vi "Configure Stamps.vi"(7 "Config Manager in":refnum<class "Config Manager Class.lvclass">, 8 "error in":errorcluster, 11 "WorkTable in":refnum<class "WorkTable Class.lvclass">) -> (0 "error out":errorcluster, 3 "WorkTable out":refnum<class "WorkTable Class.lvclass">)   [LabVIEW 2011, in "WorkTable Class.lvclass"]
uses:
  WorkTable Class.lvclass
  Config Manager Class/Config Manager Class.lvclass
  Config Manager Class/Type Definitions/Manifold Channel Types.ctl
  Type Definitions/Worktable_Stamps.ctl
  Type Definitions/Worktable_Stamp.ctl
  Utils/Type Definitions/Position_Orientation.ctl
  Vec3d Class/Vec3d Class.lvclass
  Orient3d Class/Orient3d Class.lvclass
  Config Manager Class/Type Definitions/Stamp Type.ctl
  Config Manager Class/Read Manifold Channel Other.vi
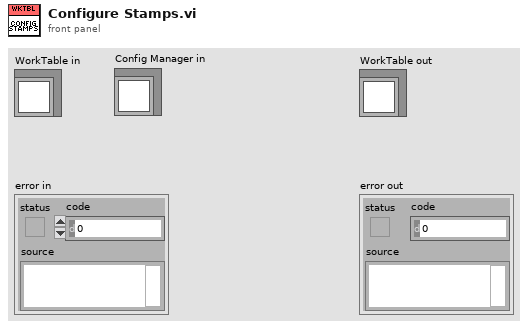
[diagram p1: front panel]
types:
  T1 = typedef "Manifold Channel Types.ctl" = enum16{"GANTRY_HEAD_OUTER", "GANTRY_HEAD_INNER", "GLUE_RESERVOIR_CHUCK", "STAMP_TOOL_CHUCK", "WEIGHT_TOOL_CHUCK"}
  T2 = typedef "Worktable_Stamps.ctl" = cluster{"Stamp Slots":T3[], "Vacuum Channel":i32}
  T3 = typedef "Worktable_Stamp.ctl" = cluster{"Stamp State":enum16{"Empty", "Populated", "Used"}, "Location/Orientation":T4, "Stamp Type":T5}
  T4 = typedef "Position_Orientation.ctl" = cluster{"Center":refnum<class "Vec3d Class.lvclass">, "Orientation":refnum<class "Orient3d Class.lvclass">}
  T5 = typedef "Stamp Type.ctl" = enum16{"Stamp 1", "Stamp 2", "Stamp 3", "Stamp 4", "Stamp 5"}
  T6 = typedef "Part Type.ctl" = enum16{"BBM", "HDI", "BARE HDI", "GLUERESERVOIR", "STAMP_1", "STAMP_2", "STAMP_3", "STAMP_4", "STAMP_5", "WEIGHT_1", "WEIGHT_2", "WEIGHT_3", "WEIGHT_4", "WEIGHT_5", "WEIGHT_6", "WEIGHT_7", "WEIGHT_8", "PICKER_TOOL", "GRABER_TOOL"}
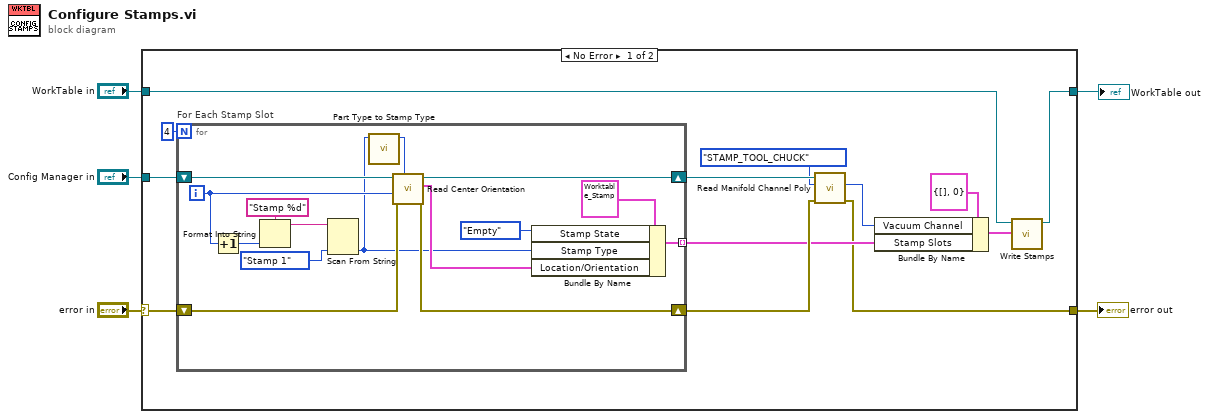
[diagram p0: block diagram]
diagram:
  n1 = case shown="No Error" "error in" {
    selector: "error in" -> [w12 w35]
    tunnel: [w6 w35] -> w2
    tunnel: [w17 w34] -> w3
    tunnel: "WorkTable in" -> [w18 w34]
    tunnel: "Config Manager in" -> [w13 _]
    frame No Error {
      n2 = for "For Each Stamp Slot" {
        N: 4 ("dimension size") -> [_]
        tunnel: [w33] -> w8 mode=indexing
        shift-right: [w26] -> w9
        shift-left: w12 -> [w27]
        shift-right: [w28] -> w11
        shift-left: w13 -> [w30]
        i -> [w25]
        n3 = Increment(x=w25) -> (x+1=w24:i32)
        n4 = Format Into String(format string="Stamp %d", w24) -> (resulting string=w22:string)  [unwired: 2 in, 1 out]
        n5 = Scan From String(input string=w22, default 1=Stamp_Type."Stamp 1" ("Stamp Type")) -> (output 1=w20:T5)  [unwired: 3 in, 3 out]
        n6 = call "Part Type to Stamp Type.vi"("Stamp Type"=w20) -> ("Part Type"=w19:T6)  [unwired: 9 in, 1 out]
        n7 = call "Read Center Orientation.vi"("Part Type"=w19, "error in"=w27, "slot"=w25, "Config Manager in"=w30) -> ("error out"=w26:errorcluster, "Location/Orientation"=w29:T4, "Config Manager out"=w28:refnum<class "Config Manager Class.lvclass">)  [unwired: 5 in]
        n8 = Bundle By Name(cluster=T3 {"Stamp State"=enum."Empty", "Location/Orientation"={"Center"=refnum, "Orientation"=refnum}, "Stamp Type"=enum."Stamp 1"} ("Stamp Slot"), "Stamp State"=enum16{"Empty", "Populated", "Used"}."Empty", "Stamp Type"=w20, "Location/Orientation"=w29) -> (w33:T3)
      }
      n9 = call-poly "Read Manifold Channel Poly.vi"("error in"=w9, "Manifold Channel Type"=Manifold_Channel_Types."STAMP_TOOL_CHUCK", "Config Manager in"=w11) -> ("error out"=w6:errorcluster, "Channel"=w7:i32)  [unwired: 6 in, 1 out]
      n10 = Bundle By Name(cluster=T2 {"Stamp Slots"=[], "Vacuum Channel"=0} ("Stamps"), "Vacuum Channel"=w7, "Stamp Slots"=w8) -> (w15:T2)
      n11 = call-dynamic "Write Stamps.vi"("Stamps"=w15, "WorkTable Class in"=w18) -> ("WorkTable Class out"=w17:refnum<class "WorkTable Class.lvclass">)  [unwired: 8 in, 1 out]
    }
    frame Error {
    }
  }
  "WorkTable out" <- w3
  "error out" <- w2
